vi "Configure 2 Wire Resistance.vi"(0 "VISA resource name":refnum<visa-resource-name>, 2 "Function":i32(ring) items=["Primary", "Secondary"], 5 "error in (no error)":errorcluster, 6 "Auto Range? (T: Auto)":bool=TRUE, 7 "Digital Filter (0: Off)":u16(ring) items=["Off", "Moving Filter", "Repeating Filter"], 8 "Custom Range (100 Ohm)":dbl=100.0 min=100.0 max=100000000.0 format="%#_6p", 9 "Digital Filter Readings (10)":i32=10, 10 "NPLC":i32(ring)=2 items=["0.001", "0.006", "0.02", "0.06", "0.1", "0.2", "0.6", "1", "2", "10", "100"]) -> (14 "VISA resource name out":refnum<visa-resource-name>, 19 "error out":errorcluster)   [LabVIEW 2024, in "Keithley 2100 Series.lvlib"]
doc: "This VI configures the instrument to measure 2-Wire Resistance.\n\nNote:\nWhen reading measurements (using the \"Data Read Single\" VI), a value of 9.9E+37 indicates overflow (i.e., an open circuit)."
uses:
  Keithley 2100 Series.lvlib
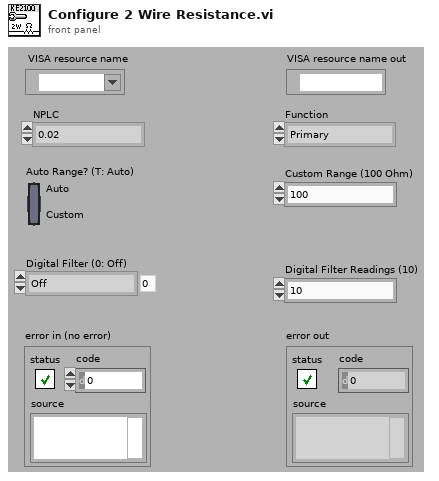
[diagram p1: front panel]
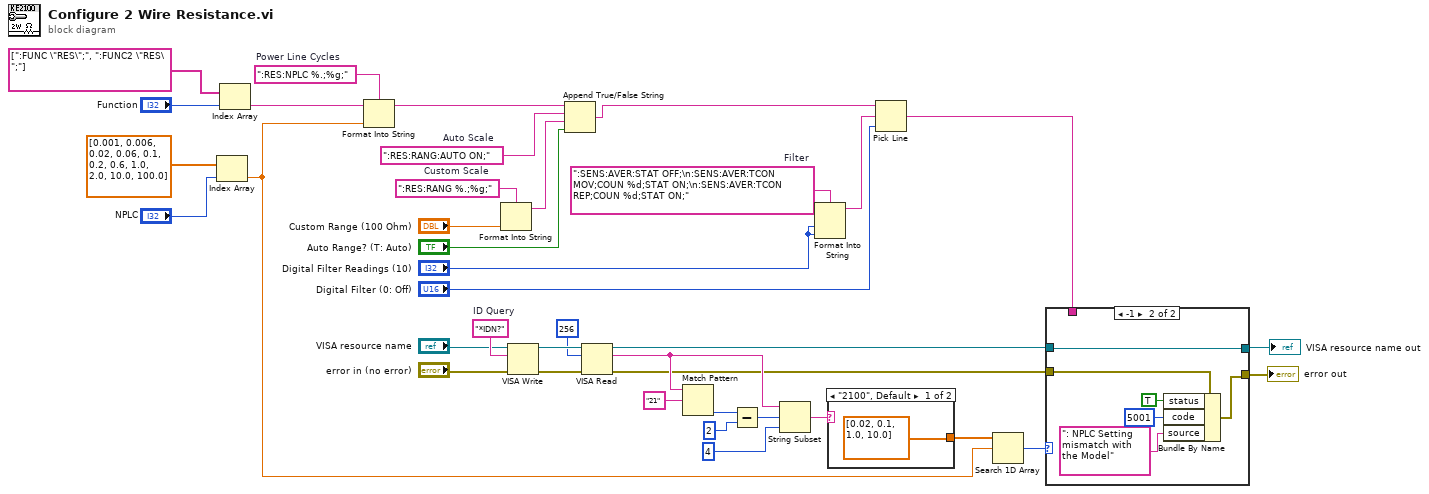
[diagram p0: block diagram]
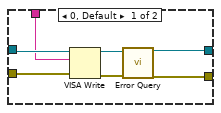
[diagram p2: hidden frame]
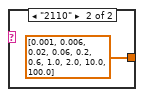
[diagram p3: hidden frame]
diagram:
  w21 = "*IDN?"  # ID Query
  w28 = ":RES:NPLC %.;%g;"  # Power Line Cycles
  w30 = ":SENS:AVER:STAT OFF;\n:SENS:AVER:TCON MOV;COUN %d;STAT ON;\n:SENS:AVER:TCON REP;COUN %d;STAT ON;"  # Filter
  w33 = ":RES:RANG:AUTO ON;"  # Auto Scale
  w35 = ":RES:RANG %.;%g;"  # Custom Scale
  n1 = Index Array(array=dbl[] [0.001, 0.006, 0.02, 0.06, 0.1, 0.2, 0.6, 1.0, 2.0, 10.0, 100.0] ("number"), index="NPLC") -> (element=w8:dbl)
  n2 = Index Array(array=string[] [":FUNC \"RES\";", ":FUNC2 \"RES\";"], index="Function") -> (element=w1:string)
  n3 = Format Into String(format string=w28, initial string=w1, w8) -> (resulting string=w37:string)  [unwired: 1 in, 1 out]
  n4 = Format Into String(format string=w35, "Custom Range (100 Ohm)") -> (resulting string=w34:string)  [unwired: 2 in, 1 out]
  n5 = VISA Write(VISA resource name="VISA resource name", write buffer=w21, error in (no error)="error in (no error)") -> (VISA resource name out=w24:refnum<visa-resource-name>, error out=w23:errorcluster)  [unwired: 1 out]
  n6 = Append True/False String(1:"Auto Range? (T: Auto)", 2:w34, 3:w33, 4:w37) -> (0:w27:string)
  n7 = VISA Read(VISA resource name=w24, byte count=u32 256, error in (no error)=w23) -> (VISA resource name out=w11:refnum<visa-resource-name>, read buffer=w15:string, error out=w10:errorcluster)  [unwired: 1 out]
  n8 = Match Pattern(string=w15, regular expression="21") -> (offset past match=w19:i32)  [unwired: 1 in, 3 out]
  n9 = Subtract(x=w19, y=2) -> (x-y=w18:i32)
  n10 = String Subset(string=w15, offset (0)=w18, length (rest)=4 ("length")) -> (substring=w14:string)
  n11 = Format Into String(format string=w30, "Digital Filter Readings (10)", "Digital Filter Readings (10)") -> (resulting string=w31:string)  [unwired: 2 in, 1 out]
  n12 = case shown="\"2100\", Default" w14 {
    tunnel: [dbl[] [0.02, 0.1, 1.0, 10.0] dbl[] [0.001, 0.006, 0.02, 0.06, 0.2, 0.6, 1.0, 2.0, 10.0, 100.0] ("number")] -> w13
    frame "2100", Default {
    }
    frame "2110" {
    }
  }
  n13 = Pick Line(string ("")=w27, multi-line string=w31, line index="Digital Filter (0: Off)") -> (output string=w9:string)
  n14 = Search 1D Array(1D array=w13, element=w8) -> (index of element=w12:i32)  [unwired: 1 in]
  n15 = case shown="-1" w12 {
    tunnel: w11 -> [w45 w53]
    tunnel: w10 -> [w44 w52]
    tunnel: [w43 w53] -> w6
    tunnel: [w42 w50] -> w7
    tunnel: w9 -> [w41 _]
    frame 0, Default {
      n16 = VISA Write(VISA resource name=w45, write buffer=w41, error in (no error)=w44) -> (VISA resource name out=w47:refnum<visa-resource-name>, error out=w46:errorcluster)  [unwired: 1 out]
      n17 = call "Error Query.vi"("VISA resource name"=w47, "error in (no error)"=w46) -> ("VISA resource name out"=w43:refnum<visa-resource-name>, "error out"=w42:errorcluster)  [unwired: 14 in, 2 out]
    }
    frame -1 {
      n18 = Bundle By Name(cluster=w52, "status"=TRUE, "code"=5001, "source"=": NPLC Setting mismatch with the Model") -> (w50:errorcluster)
    }
  }
  "error out" <- w7
  "VISA resource name out" <- w6
